vi "Wait.vi"(6 "WaitTimeout_ms (-1 indefinite)":i32=-1, 8 "error in (no error)":errorcluster, 11 "HttpDownloadTask in":T1) -> (0 "error out":errorcluster, 1 "Canceled":bool, 3 "HttpDownloadTask out":T1, 4 "Wait Timed out":bool)   [LabVIEW 2018, in "HttpClient_NET.lvlib" / "HttpDownloadTask.lvclass"]
uses:
  HttpDownloadTask.lvclass
  Types/DownloadTask_ref.ctl
  HttpDownloadTask.lvclass/HttpDownloadTask.ctl
  Accessors/Read HttpContent out.vi
  HttpContent/HttpContent.lvclass
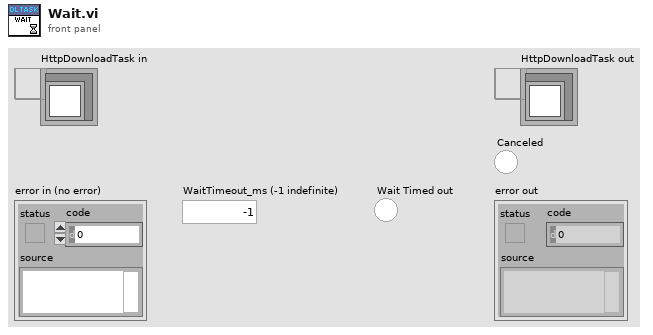
[diagram p1: front panel]
types:
  T1 = typedef "HttpClient_NET.lvlib/HttpDownloadTask.lvclass/DownloadTask_ref.ctl" = refnum<data-value>
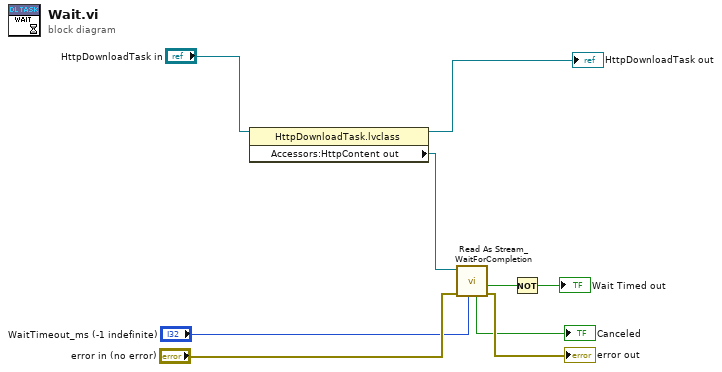
[diagram p0: block diagram]
diagram:
  n1 = property class="HttpDownloadTask.lvclass"(reference="HttpDownloadTask in") -> (reference out=→"HttpDownloadTask out":T1, "Accessors:HttpContent out"=w7:refnum<class "HttpContent.lvclass">)  [unwired: 1 in, 1 out]
  n2 = call "Read As Stream_WaitForCompletion.vi"("millisecondsTimeout (-1 indefinite)"="WaitTimeout_ms (-1 indefinite)", "error in (no error)"="error in (no error)", "HttpContent in"=w7) -> ("error out"=→"error out":errorcluster, "IsCompleted"=w3:bool, "Canceled"=→"Canceled":bool)  [unwired: 5 in, 1 out]
  n3 = Not(x=w3) -> (.not. x?=→"Wait Timed out":bool)
